vi "Drag Panel-Get Window Name.vi"(8 "error in":errorcluster, 11 "VI Refnum In":refnum<vi>) -> (0 "error out":errorcluster, 2 "Window Name":string, 3 "VI Refnum Out":refnum<vi>)   [LabVIEW 2018]
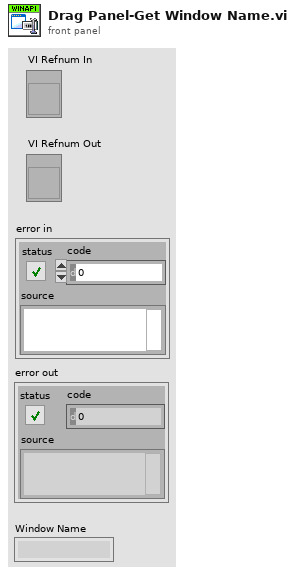
[diagram p1: front panel]
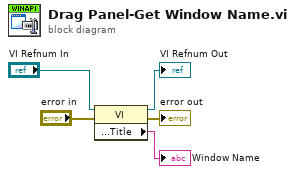
[diagram p0: block diagram]
diagram:
  n1 = property class="VI"(reference="VI Refnum In", error in="error in") -> (reference out=→"VI Refnum Out":refnum<vi>, error out=→"error out":errorcluster, "Front Panel.Title"=→"Window Name":string)
